vi "Convert 4-port S to T.vi"() -> ()   [LabVIEW 2020]
uses:
  <vilib>/Analysis/Matrix/NI_Matrix.lvlib
  <vilib>/Analysis/NI_AALBase.lvlib
  <vilib>/addons/HF Network Analysis/NI_HFNetworkAnalysis.lvlib
  <vilib>/Analysis/Matrix/Numeric/Conversions/Array To Matrix - RA2.vi
  <vilib>/Analysis/baseanly.llb/Real A x B.vi
  <vilib>/Analysis/Matrix/Numeric/Subtract/Subtract - RM,RM.vi
  <vilib>/Analysis/Matrix/Numeric/Conversions/Matrix To Array - RM.vi
  <vilib>/Analysis/baseanly.llb/Real Inverse Matrix.vi
panel:
  out "Complex 2D Array":cdb[][][](array[numeric])
  in  "Ring":u16(ring) items=["denumerator", "T11", "T12", "T13", "T14", "T21", "T22", "T23", "T24", "T31", "T32", "T33", "T34", "T41", "T42", "T43", "T44"]
  out "Array":cdb[][][](array[numeric])
  in  "Parameters In (2D)":cdb[][](array[numeric]) format="%.3f"
  # "11 \n12 \n13 \n14\n21 \n22 \n23 \n24\n31 \n32 \n33 \n34\n41 \n42 \n43 \n44"
  # "11 12 13 14\n21 22 23 24\n31 32 33 34\n41 42 43 44"
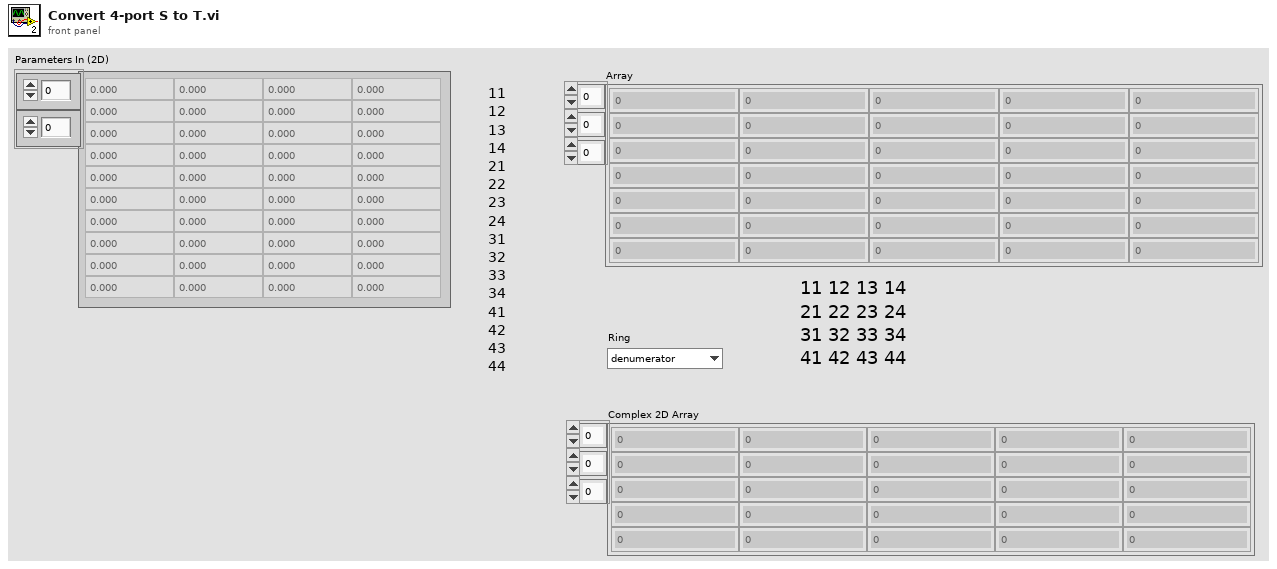
[diagram p1: front panel]
types:
  T1 = typedef "LVStringsAndValuesArrayTypeDef_U16.ctl" = cluster{"String":string, "Value":u16}[]
  T2 = typedef "NI_Matrix.lvlib/RealMatrix.ctl" = dbl[][]
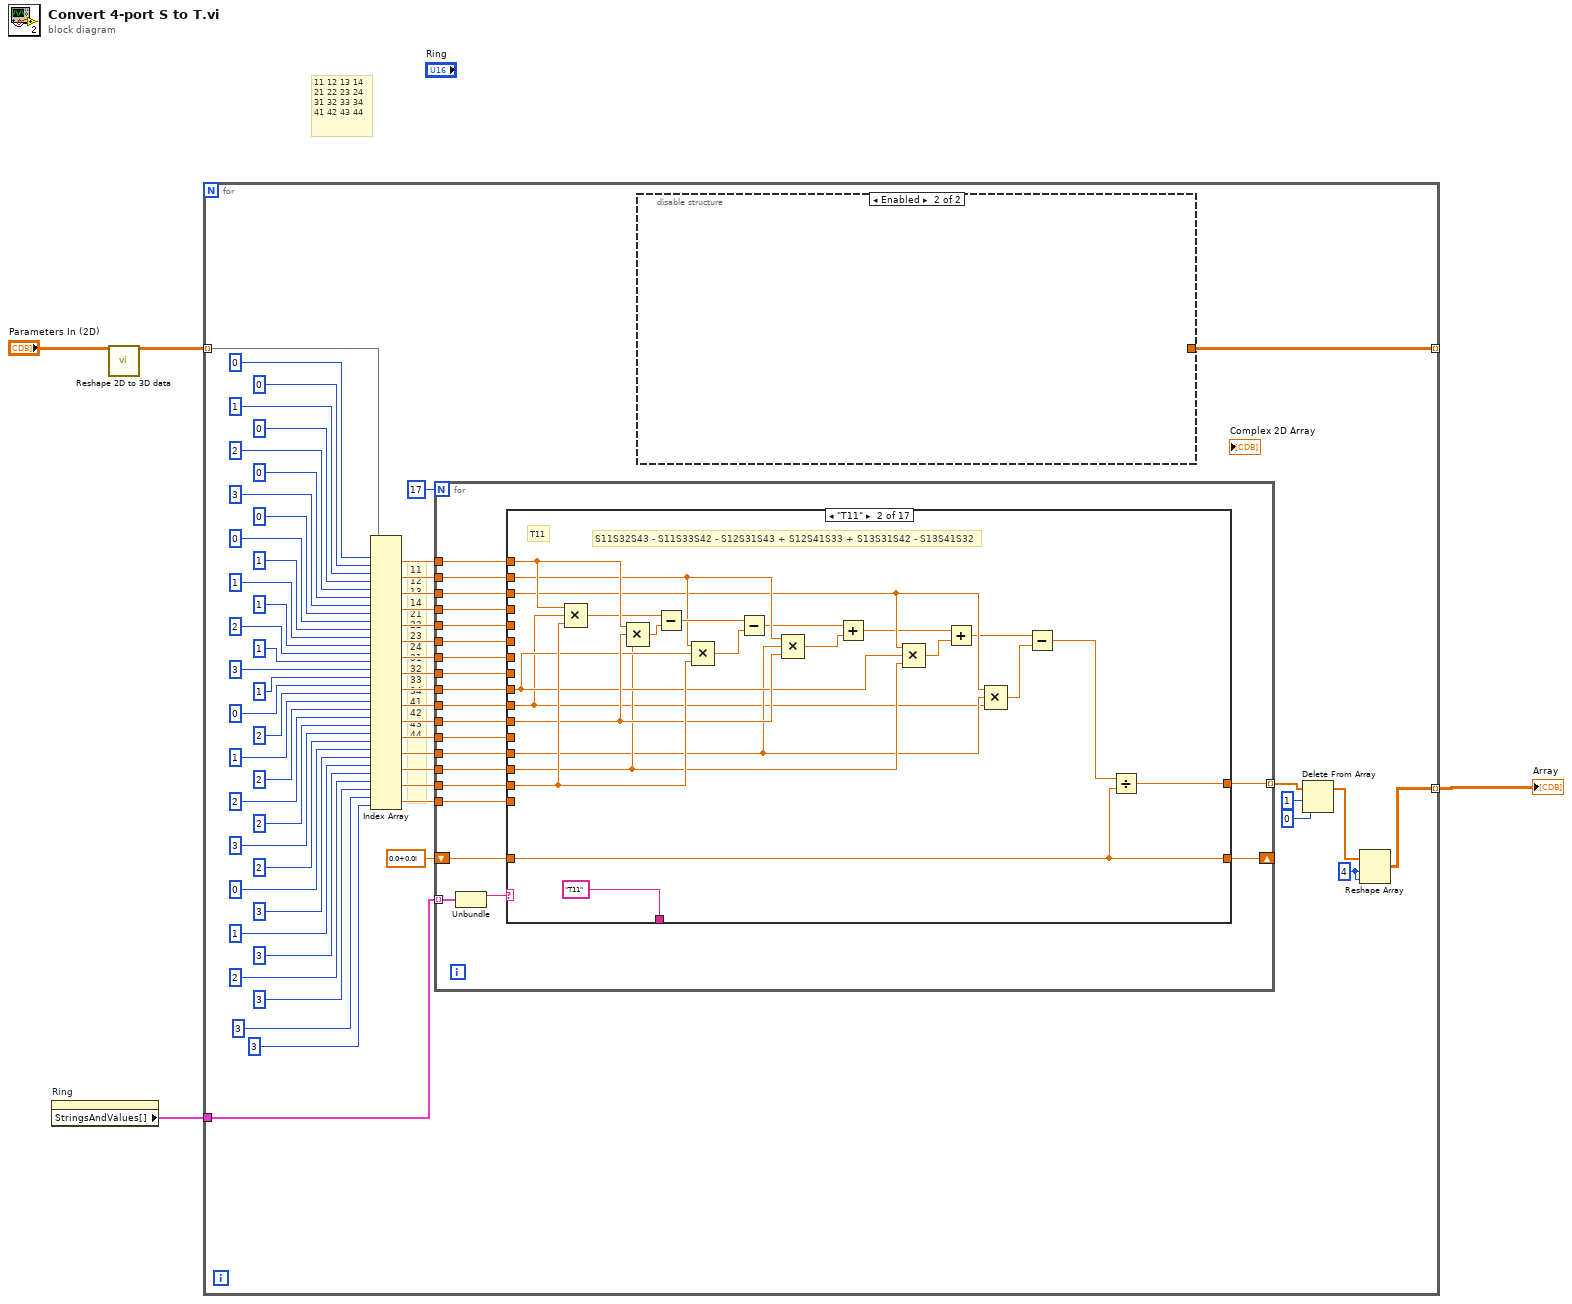
[diagram p0: block diagram]
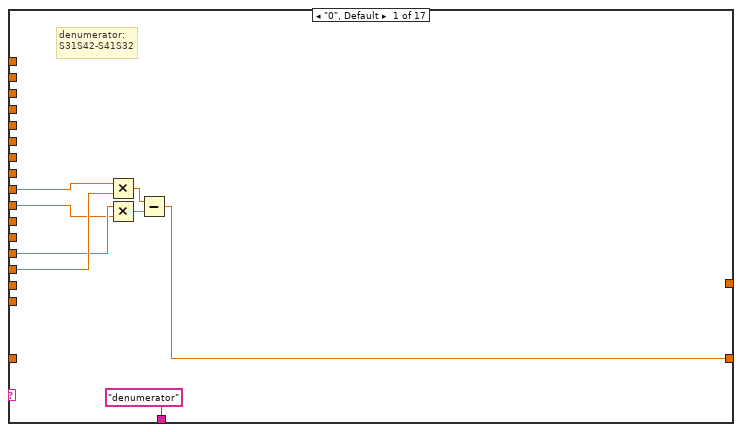
[diagram p2: hidden frame]
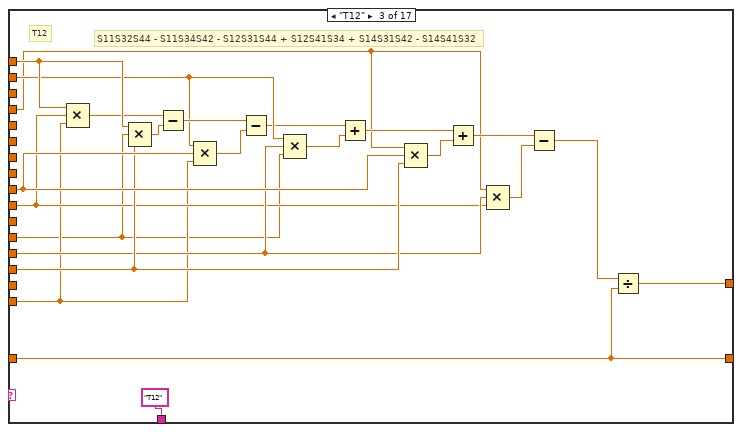
[diagram p3: hidden frame]
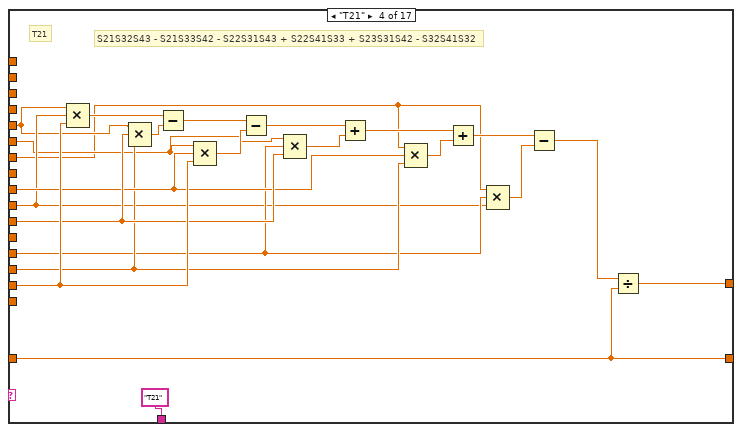
[diagram p4: hidden frame]
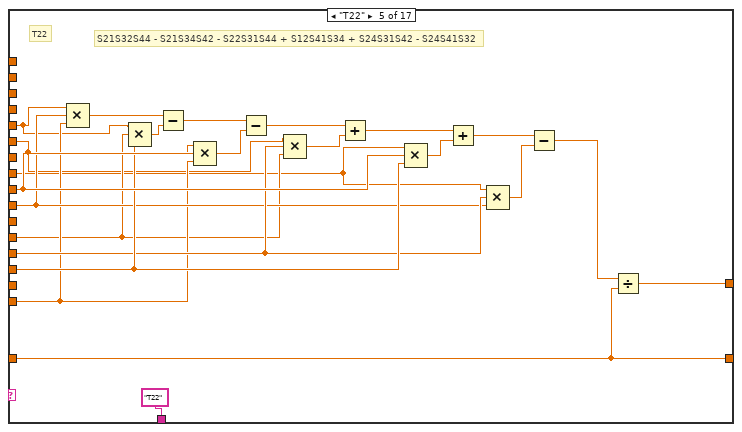
[diagram p5: hidden frame]
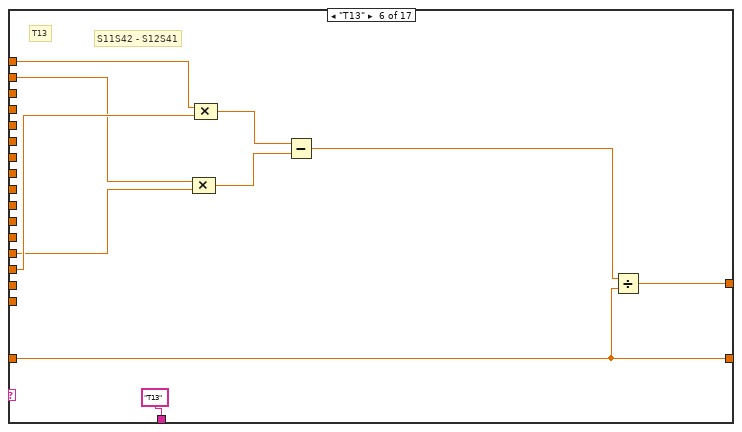
[diagram p6: hidden frame]
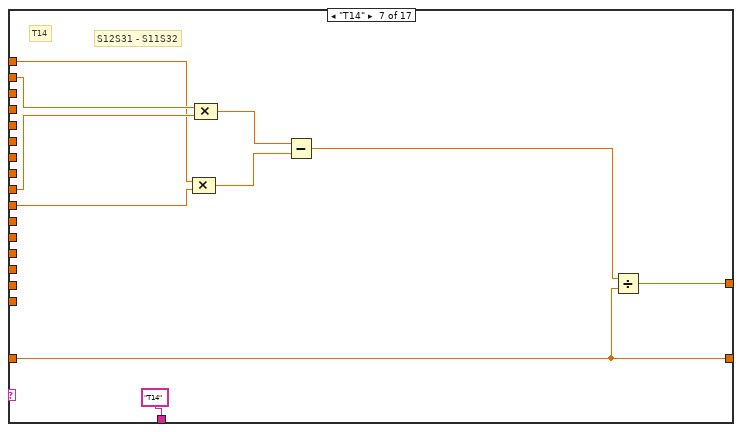
[diagram p7: hidden frame]
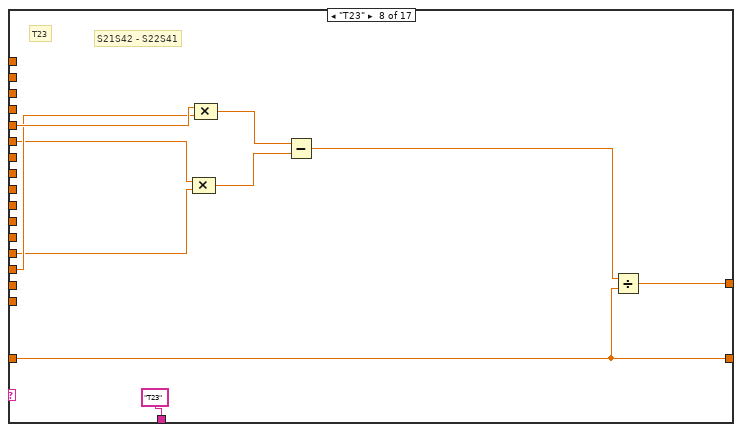
[diagram p8: hidden frame]
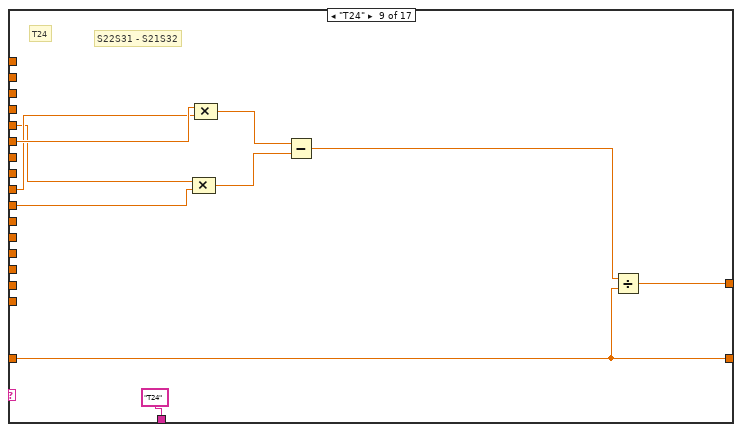
[diagram p9: hidden frame]
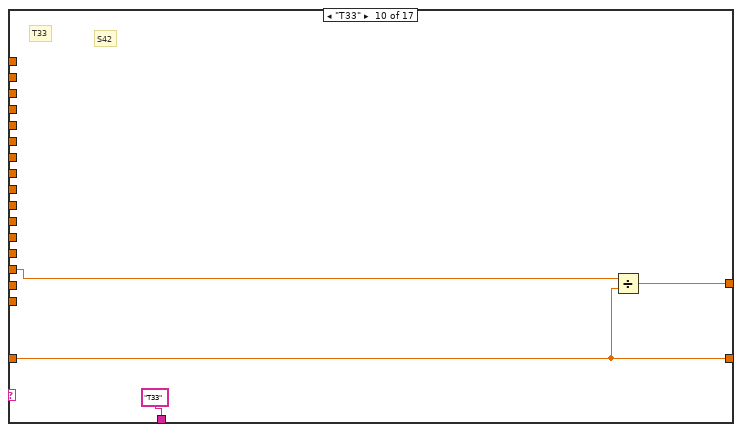
[diagram p10: hidden frame]
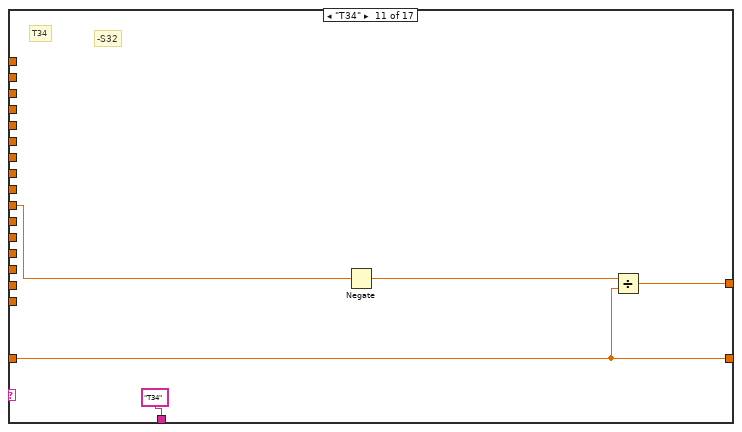
[diagram p11: hidden frame]
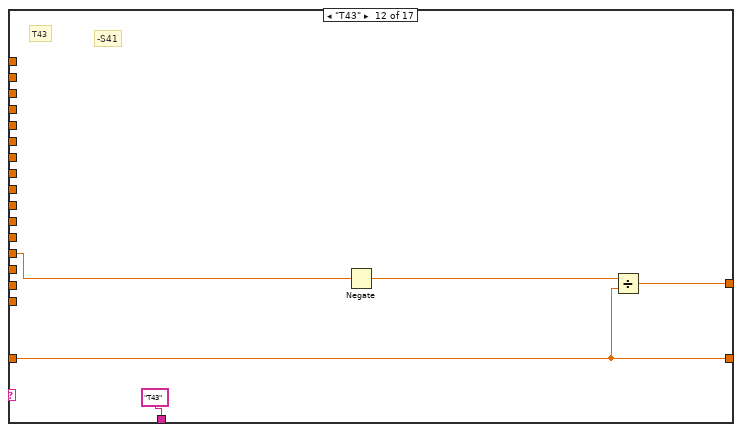
[diagram p12: hidden frame]
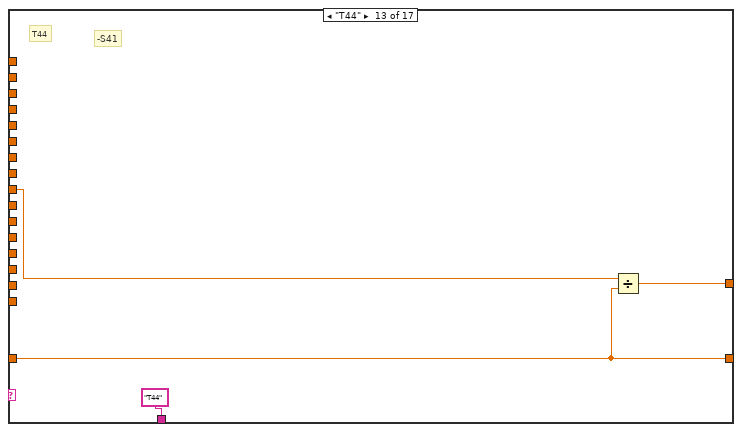
[diagram p13: hidden frame]
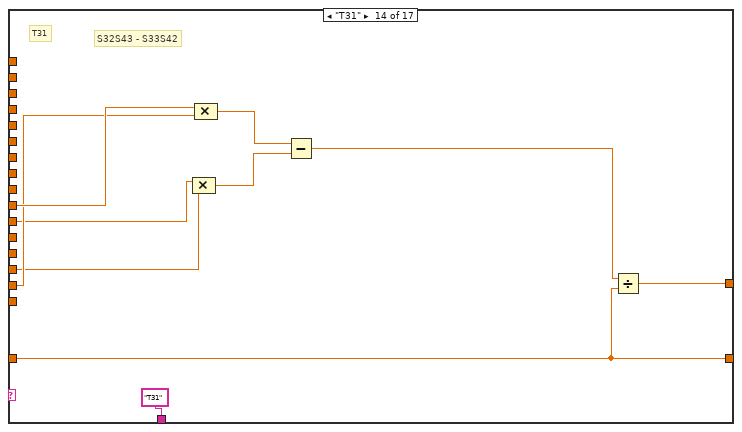
[diagram p14: hidden frame]
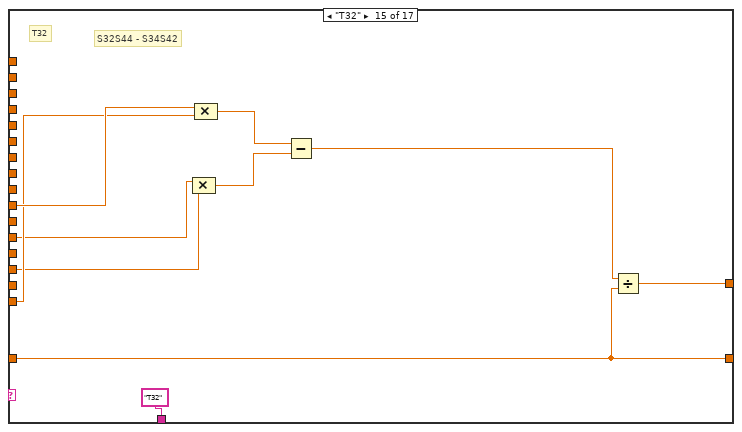
[diagram p15: hidden frame]
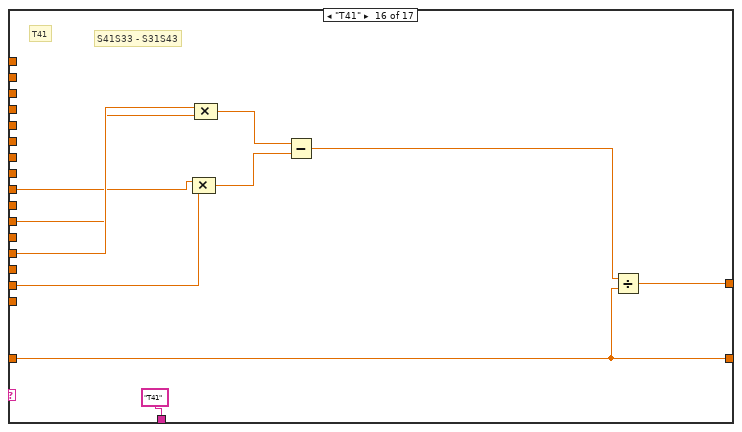
[diagram p16: hidden frame]
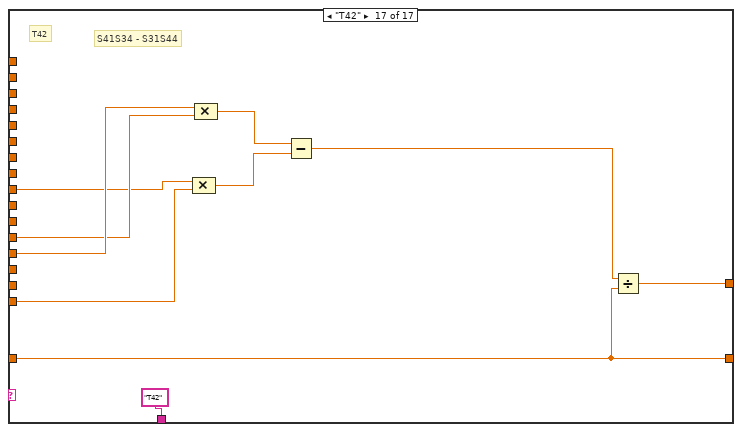
[diagram p17: hidden frame]
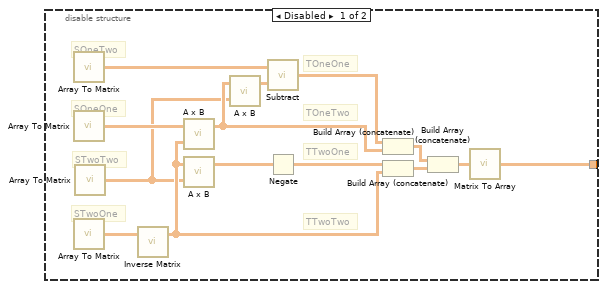
[diagram p18: hidden frame]
diagram:
  # "11 12 13 14\n21 22 23 24\n31 32 33 34\n41 42 43 44"
  n1 = property on="Ring" class="Ring (strict)"() -> ("StringsAndValues[]"=w1:T1)  [unwired: 2 in, 2 out]
  n2 = call <vilib>:"Reshape 2D to 3D data.vi"("Parameters In (2D)"="Parameters In (2D)") -> ("Parameters Out (3D)"=w4:cdb[][][])  [unwired: 13 in, 1 out]
  n3 = for {
    tunnel: w4 -> [w62] mode=indexing
    tunnel: [w63] -> _ mode=indexing
    tunnel: [w7] -> w2 mode=indexing
    tunnel: w1 -> [w5]
    w6 = 4 ("dimension size")
    # "11 \n12 \n13 \n14\n21 \n22 \n23 \n24\n31 \n32 \n33 \n34\n41 \n42 \n43 \n44"
    n4 = Index Array(array=w62, index (row) #1=0 ("index (row)"), index (col) #1=0 ("disabled index (col)"), index (row) #2=1 ("index (row)"), index (col) #2=0 ("disabled index (col)"), index (row) #3=2 ("index (row)"), index (col) #3=0 ("disabled index (col)"), index (row) #4=3 ("index (row)"), index (col) #4=0 ("disabled index (col)"), index (row) #5=0 ("index (row)"), index (col) #5=1 ("disabled index (col)"), index (row) #6=1 ("index (row)"), index (col) #6=1 ("disabled index (col)"), index (row) #7=2 ("index (row)"), index (col) #7=1 ("disabled index (col)"), index (row) #8=3 ("index (row)"), index (col) #8=1 ("disabled index (col)"), index (row) #9=0 ("index (row)"), index (col) #9=2 ("disabled index (col)"), index (row) #10=1 ("index (row)"), index (col) #10=2 ("disabled index (col)"), index (row) #11=2 ("index (row)"), index (col) #11=2 ("disabled index (col)"), index (row) #12=3 ("index (row)"), index (col) #12=2 ("disabled index (col)"), index (row) #13=0 ("index (row)"), index (col) #13=3 ("disabled index (col)"), index (row) #14=1 ("index (row)"), index (col) #14=3 ("disabled index (col)"), index (row) #15=2 ("index (row)"), index (col) #15=3 ("disabled index (col)"), index (row) #16=3 ("index (row)"), index (col) #16=3 ("disabled index (col)")) -> (element #1=w24:cdb, element #2=w21:cdb, element #3=w20:cdb, element #4=w16:cdb, element #5=w15:cdb, element #6=w14:cdb, element #7=w13:cdb, element #8=w12:cdb, element #9=w29:cdb, element #10=w26:cdb, element #11=w22:cdb, element #12=w17:cdb, element #13=w27:cdb, element #14=w28:cdb, element #15=w23:cdb, element #16=w18:cdb)
    n5 = for {
      N: 17 -> [_]
      tunnel: w29 -> [w84]
      tunnel: w28 -> [w83]
      tunnel: w27 -> [w82]
      tunnel: w26 -> [w81]
      shift-right: [w80] -> _
      shift-left: cdb 0.0+0.0i -> [w79]
      tunnel: w24 -> [w78]
      tunnel: w23 -> [w77]
      tunnel: w22 -> [w76]
      tunnel: w21 -> [w75]
      tunnel: w20 -> [w74]
      tunnel: [w73] -> w11 mode=indexing
      tunnel: w18 -> [w72]
      tunnel: w17 -> [w71]
      tunnel: w16 -> [w70]
      tunnel: w15 -> [w69]
      tunnel: w14 -> [w68]
      tunnel: w13 -> [w67]
      tunnel: w12 -> [w66]
      tunnel: w5 -> [w64] mode=indexing
      n6 = Unbundle(w64) -> ("String"=w65:string)  [unwired: 1 out]
      n7 = case shown="\"T11\"" w65 {
        tunnel: w84 -> [w90 w106 w131 w154 w179 _ w198 _ w218 _ _ _ w240 _ _ w265 w275]
        tunnel: w83 -> [w89 w105 w130 w153 w178 w189 _ w208 _ w226 _ _ _ w244 w254 _ _]
        tunnel: w82 -> [w88 w103 w129 w152 w177 w187 _ w206 _ _ _ w235 _ _ _ w267 w277]
        tunnel: w81 -> [w87 w102 w128 w151 w176 _ w196 _ w216 _ w231 _ _ w247 w257 _ _]
        tunnel: [w86 w109 w133 w156 w180 w191 w202 w212 w222 w228 w233 w238 w242 w250 w260 w270 w280] -> w80
        tunnel: w79 -> [_ w109 w133 w156 w180 w191 w202 w212 w222 w228 w233 w238 w242 w250 w260 w270 w280]
        tunnel: w78 -> [_ w115 w138 _ _ w194 w197 _ _ _ _ _ _ _ _ _ _]
        tunnel: w77 -> [_ w114 _ w161 _ _ _ _ _ _ _ _ _ w246 _ w264 _]
        tunnel: w76 -> [_ w107 _ w155 _ _ _ _ _ _ _ _ _ w245 _ w266 _]
        tunnel: w75 -> [_ w108 w132 _ _ w188 w199 _ _ _ _ _ _ _ _ _ _]
        tunnel: w74 -> [_ w104 _ _ _ _ _ _ _ _ _ _ _ _ _ _ _]
        tunnel: [_ w94 w120 w143 w168 w190 w201 w211 w221 w227 w232 w237 w241 w249 w259 w269 w279] -> w73
        tunnel: w72 -> [_ _ w119 _ w167 _ _ _ _ _ _ _ _ _ w256 _ w274]
        tunnel: w71 -> [_ _ w118 _ w166 _ _ _ _ _ _ _ _ _ w255 _ w276]
        tunnel: w70 -> [_ _ w117 _ _ _ _ _ _ _ _ _ _ _ _ _ _]
        tunnel: w69 -> [_ _ _ w142 w165 _ _ w209 w217 _ _ _ _ _ _ _ _]
        tunnel: w68 -> [_ _ _ w141 w164 _ _ w207 w219 _ _ _ _ _ _ _ _]
        tunnel: w67 -> [_ _ _ w140 _ _ _ _ _ _ _ _ _ _ _ _ _]
        tunnel: w66 -> [_ _ _ _ w163 _ _ _ _ _ _ _ _ _ _ _ _]
        tunnel: ["denumerator" "T11" "T12" "T21" "T22" "T13" "T14" "T23" "T24" "T33" "T34" "T43" "T44" "T31" "T32" "T41" "T42"] -> _
        frame "0", Default {
          # "denumerator:\nS31S42-S41S32"
          n8 = Multiply(x=w90, y=w89) -> (x*y=w92:cdb)
          n9 = Multiply(x=w88, y=w87) -> (x*y=w91:cdb)
          n10 = Subtract(x=w92, y=w91) -> (x-y=w86:cdb)
        }
        frame "T11" {
          # "T11"
          # "S11S32S43 - S11S33S42 - S12S31S43 + S12S41S33 + S13S31S42 - S13S41S32"
          n11 = Compound Arithmetic op=MULTIPLY(w115, w102, w114) -> (w110:cdb)
          n12 = Compound Arithmetic op=MULTIPLY(w115, w107, w105) -> (w113:cdb)
          n13 = Subtract(x=w110, y=w113) -> (x-y=w111:cdb)
          n14 = Compound Arithmetic op=MULTIPLY(w108, w106, w114) -> (w112:cdb)
          n15 = Subtract(x=w111, y=w112) -> (x-y=w97:cdb)
          n16 = Compound Arithmetic op=MULTIPLY(w108, w103, w107) -> (w98:cdb)
          n17 = Add(x=w97, y=w98) -> (x+y=w99:cdb)
          n18 = Compound Arithmetic op=MULTIPLY(w104, w106, w105) -> (w100:cdb)
          n19 = Add(x=w99, y=w100) -> (x+y=w101:cdb)
          n20 = Compound Arithmetic op=MULTIPLY(w104, w103, w102) -> (w96:cdb)
          n21 = Subtract(x=w101, y=w96) -> (x-y=w95:cdb)
          n22 = Divide(x=w95, y=w109) -> (x/y=w94:cdb)
        }
        frame "T12" {
          # "T12"
          # "S11S32S44 - S11S34S42 - S12S31S44 + S12S41S34 + S14S31S42 - S14S41S32"
          n23 = Compound Arithmetic op=MULTIPLY(w138, w128, w119) -> (w134:cdb)
          n24 = Compound Arithmetic op=MULTIPLY(w138, w118, w130) -> (w137:cdb)
          n25 = Subtract(x=w134, y=w137) -> (x-y=w135:cdb)
          n26 = Compound Arithmetic op=MULTIPLY(w132, w131, w119) -> (w136:cdb)
          n27 = Subtract(x=w135, y=w136) -> (x-y=w123:cdb)
          n28 = Compound Arithmetic op=MULTIPLY(w132, w129, w118) -> (w124:cdb)
          n29 = Add(x=w123, y=w124) -> (x+y=w125:cdb)
          n30 = Compound Arithmetic op=MULTIPLY(w117, w131, w130) -> (w126:cdb)
          n31 = Add(x=w125, y=w126) -> (x+y=w127:cdb)
          n32 = Compound Arithmetic op=MULTIPLY(w117, w129, w128) -> (w122:cdb)
          n33 = Subtract(x=w127, y=w122) -> (x-y=w121:cdb)
          n34 = Divide(x=w121, y=w133) -> (x/y=w120:cdb)
        }
        frame "T21" {
          # "T21"
          # "S21S32S43 - S21S33S42 - S22S31S43 + S22S41S33 + S23S31S42 - S32S41S32"
          n35 = Compound Arithmetic op=MULTIPLY(w142, w151, w161) -> (w157:cdb)
          n36 = Compound Arithmetic op=MULTIPLY(w142, w155, w153) -> (w160:cdb)
          n37 = Subtract(x=w157, y=w160) -> (x-y=w158:cdb)
          n38 = Compound Arithmetic op=MULTIPLY(w141, w154, w161) -> (w159:cdb)
          n39 = Subtract(x=w158, y=w159) -> (x-y=w146:cdb)
          n40 = Compound Arithmetic op=MULTIPLY(w141, w152, w155) -> (w147:cdb)
          n41 = Add(x=w146, y=w147) -> (x+y=w148:cdb)
          n42 = Compound Arithmetic op=MULTIPLY(w140, w154, w153) -> (w149:cdb)
          n43 = Add(x=w148, y=w149) -> (x+y=w150:cdb)
          n44 = Compound Arithmetic op=MULTIPLY(w140, w152, w151) -> (w145:cdb)
          n45 = Subtract(x=w150, y=w145) -> (x-y=w144:cdb)
          n46 = Divide(x=w144, y=w156) -> (x/y=w143:cdb)
        }
        frame "T22" {
          # "T22"
          # "S21S32S44 - S21S34S42 - S22S31S44 + S12S41S34 + S24S31S42 - S24S41S32"
          n47 = Compound Arithmetic op=MULTIPLY(w165, w176, w167) -> (w181:cdb)
          n48 = Compound Arithmetic op=MULTIPLY(w165, w166, w178) -> (w184:cdb)
          n49 = Subtract(x=w181, y=w184) -> (x-y=w182:cdb)
          n50 = Compound Arithmetic op=MULTIPLY(w164, w179, w167) -> (w183:cdb)
          n51 = Subtract(x=w182, y=w183) -> (x-y=w171:cdb)
          n52 = Compound Arithmetic op=MULTIPLY(w164, w177, w166) -> (w172:cdb)
          n53 = Add(x=w171, y=w172) -> (x+y=w173:cdb)
          n54 = Compound Arithmetic op=MULTIPLY(w163, w179, w178) -> (w174:cdb)
          n55 = Add(x=w173, y=w174) -> (x+y=w175:cdb)
          n56 = Compound Arithmetic op=MULTIPLY(w163, w177, w176) -> (w170:cdb)
          n57 = Subtract(x=w175, y=w170) -> (x-y=w169:cdb)
          n58 = Divide(x=w169, y=w180) -> (x/y=w168:cdb)
        }
        frame "T13" {
          # "T13"
          # "S11S42 - S12S41"
          n59 = Compound Arithmetic op=MULTIPLY(w188, w187) -> (w193:cdb)
          n60 = Compound Arithmetic op=MULTIPLY(w194, w189) -> (w192:cdb)
          n61 = Subtract(x=w192, y=w193) -> (x-y=w186:cdb)
          n62 = Divide(x=w186, y=w191) -> (x/y=w190:cdb)
        }
        frame "T14" {
          # "T14"
          # "S12S31 - S11S32"
          n63 = Compound Arithmetic op=MULTIPLY(w197, w196) -> (w204:cdb)
          n64 = Compound Arithmetic op=MULTIPLY(w199, w198) -> (w203:cdb)
          n65 = Subtract(x=w203, y=w204) -> (x-y=w200:cdb)
          n66 = Divide(x=w200, y=w202) -> (x/y=w201:cdb)
        }
        frame "T23" {
          # "T23"
          # "S21S42 - S22S41"
          n67 = Compound Arithmetic op=MULTIPLY(w207, w206) -> (w214:cdb)
          n68 = Compound Arithmetic op=MULTIPLY(w209, w208) -> (w213:cdb)
          n69 = Subtract(x=w213, y=w214) -> (x-y=w210:cdb)
          n70 = Divide(x=w210, y=w212) -> (x/y=w211:cdb)
        }
        frame "T24" {
          # "T24"
          # "S22S31 - S21S32"
          n71 = Compound Arithmetic op=MULTIPLY(w217, w216) -> (w224:cdb)
          n72 = Compound Arithmetic op=MULTIPLY(w219, w218) -> (w223:cdb)
          n73 = Subtract(x=w223, y=w224) -> (x-y=w220:cdb)
          n74 = Divide(x=w220, y=w222) -> (x/y=w221:cdb)
        }
        frame "T33" {
          # "T33"
          # "S42"
          n75 = Divide(x=w226, y=w228) -> (x/y=w227:cdb)
        }
        frame "T34" {
          # "T34"
          # "-S32"
          n76 = Negate(x=w231) -> (-x=w230:cdb)
          n77 = Divide(x=w230, y=w233) -> (x/y=w232:cdb)
        }
        frame "T43" {
          # "T43"
          # "-S41"
          n78 = Negate(x=w235) -> (-x=w236:cdb)
          n79 = Divide(x=w236, y=w238) -> (x/y=w237:cdb)
        }
        frame "T44" {
          # "T44"
          # "-S41"
          n80 = Divide(x=w240, y=w242) -> (x/y=w241:cdb)
        }
        frame "T31" {
          # "T31"
          # "S32S43 - S33S42"
          n81 = Compound Arithmetic op=MULTIPLY(w245, w244) -> (w252:cdb)
          n82 = Compound Arithmetic op=MULTIPLY(w247, w246) -> (w251:cdb)
          n83 = Subtract(x=w251, y=w252) -> (x-y=w248:cdb)
          n84 = Divide(x=w248, y=w250) -> (x/y=w249:cdb)
        }
        frame "T32" {
          # "T32"
          # "S32S44 - S34S42"
          n85 = Compound Arithmetic op=MULTIPLY(w255, w254) -> (w262:cdb)
          n86 = Compound Arithmetic op=MULTIPLY(w257, w256) -> (w261:cdb)
          n87 = Subtract(x=w261, y=w262) -> (x-y=w258:cdb)
          n88 = Divide(x=w258, y=w260) -> (x/y=w259:cdb)
        }
        frame "T41" {
          # "T41"
          # "S41S33 - S31S43"
          n89 = Compound Arithmetic op=MULTIPLY(w265, w264) -> (w272:cdb)
          n90 = Compound Arithmetic op=MULTIPLY(w267, w266) -> (w271:cdb)
          n91 = Subtract(x=w271, y=w272) -> (x-y=w268:cdb)
          n92 = Divide(x=w268, y=w270) -> (x/y=w269:cdb)
        }
        frame "T42" {
          # "T42"
          # "S41S34 - S31S44"
          n93 = Compound Arithmetic op=MULTIPLY(w275, w274) -> (w282:cdb)
          n94 = Compound Arithmetic op=MULTIPLY(w277, w276) -> (w281:cdb)
          n95 = Subtract(x=w281, y=w282) -> (x-y=w278:cdb)
          n96 = Divide(x=w278, y=w280) -> (x/y=w279:cdb)
        }
      }
    }
    n97 = disable-structure shown="Enabled" {
      disable-tunnel: [w283 _] -> w63
      frame Disabled {
        # "TTwoOne"
        # "TOneTwo"
        # "TOneOne"
        # "TTwoTwo"
        # "STwoTwo"
        # "STwoOne"
        # "SOneTwo"
        # "SOneOne"
        n98 = call-poly <vilib>:"Array To Matrix.vi"() -> ("Real Matrix"=w294:T2)  [unwired: 1 in]
        n99 = call-poly <vilib>:"Array To Matrix.vi"() -> ("Real Matrix"=w295:T2)  [unwired: 1 in]
        n100 = call-poly <vilib>:"Array To Matrix.vi"() -> ("Real Matrix"=w296:T2)  [unwired: 1 in]
        n101 = call-poly <vilib>:"Array To Matrix.vi"() -> ("Real Matrix"=w285:T2)  [unwired: 1 in]
        n102 = call-poly <vilib>:"Inverse Matrix.vi"("Input Matrix"=w296) -> ("Inverse Matrix"=w286:T2)  [unwired: 1 in, 1 out]
        n103 = call-poly <vilib>:"A x B.vi"("B"=w286, "A"=w295) -> ("A x B"=w289:T2)  [unwired: 1 out]
        n104 = call-poly <vilib>:"A x B.vi"("B"=w285, "A"=w286) -> ("A x B"=w288:T2)  [unwired: 1 out]
        n105 = call-poly <vilib>:"A x B.vi"("B"=w285, "A"=w289) -> ("A x B"=w293:T2)  [unwired: 1 out]
        n106 = call-poly <vilib>:"Subtract.vi"("Real Matrix B"=w293, "Real Matrix A"=w294) -> ("A - B"=w290:T2)
        n107 = Negate(x=w288) -> (-x=w287:T2)
        n108 = Build Array (concatenate)(w290, w289) -> (w292:T2)
        n109 = Build Array (concatenate)(w287, w286) -> (w291:T2)
        n110 = Build Array (concatenate)(w292, w291) -> (w284:T2)
        n111 = call-poly <vilib>:"Matrix To Array.vi"("Real Matrix"=w284) -> ("Real 2D Array"=w283:dbl[][])
      }
      frame Enabled {
      }
    }
    n112 = Delete From Array(array=w11, length=1, index=0) -> (array with subset deleted=w8:cdb[])  [unwired: 1 out]
    n113 = Reshape Array(w8, w6, w6) -> (w7:cdb[][])
  }
  "Array" <- w2
